vi "Initialize Dropbox Folder.vi"(1 "Computer:":string(combo)="Jeevan-Laptop2") -> (0 "Dropbox Directory":string)   [LabVIEW 2011]
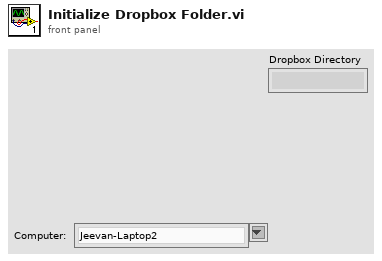
[diagram p1: front panel]
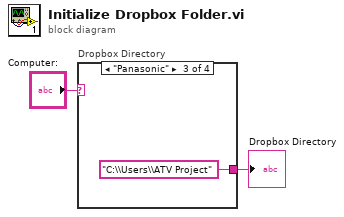
[diagram p0: block diagram]
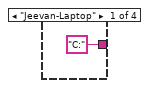
[diagram p2: hidden frame]
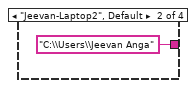
[diagram p3: hidden frame]
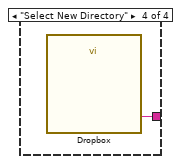
[diagram p4: hidden frame]
diagram:
  n1 = case "Dropbox Directory" shown="\"Panasonic\"" "Computer:" {
    tunnel: ["C:" ("Directory") "C:\\Users\\Jeevan Anga" ("Drive (with colon) :") "C:\\Users\\ATV Project" ("Drive (with colon) :") w6] -> w2
    frame "Jeevan-Laptop" {
    }
    frame "Jeevan-Laptop2", Default {
    }
    frame "Panasonic" {
    }
    frame "Select New Directory" {
      n2 = call "Dropbox"() -> ("Drive (with colon) :"=w6:string)  [unwired: 17 in, 2 out]
    }
  }
  "Dropbox Directory" <- w2
